vi "tlc_Timing Module Unit Test.vi"() -> ()   [LabVIEW 2010]
uses:
  Controls/tlc_Cue_Information.ctl
  Controls/channel.ctl
  tlc_Timing Module Unit Test States.ctl
  tlc_Timing Command Control.ctl
panel:
  out "Follow Time (s)":dbl format="%.2f"
  out "Fade Time (s)":dbl format="%.2f"
  out "Wait Time (s)":dbl format="%.2f"
  in  "Cue Input":T1 {"Channels"."Intensität" min=0.0 max=100.0 step=1.0 format="%#.0f"}
  # "Measured Test Values"
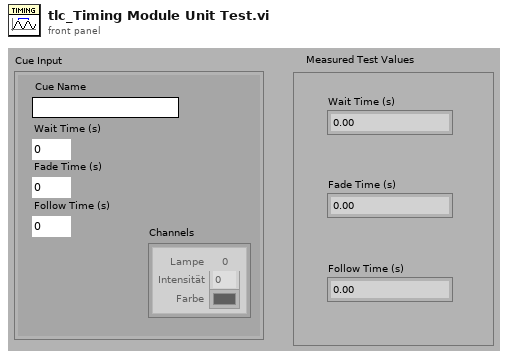
[diagram p1: front panel]
types:
  T1 = typedef "tlc_Cue_Information.ctl" = cluster{"Cue Name":string, "Wait Time (s)":u32, "Fade Time (s)":u32, "Follow Time (s)":u32, "Channels":T2[][]}
  T2 = typedef "channel.ctl" = cluster{"Intensität":dbl, " Farbe":u32, "Channel":i32}
  T3 = typedef "tlc_Timing Module Unit Test States.ctl" = enum16{"Begin Play", "Wait Time", "Fade Time", "Follow Time", "End Play"}
  T4 = typedef "tlc_Timing Command Control.ctl" = enum16{"Start", "Check Time"}
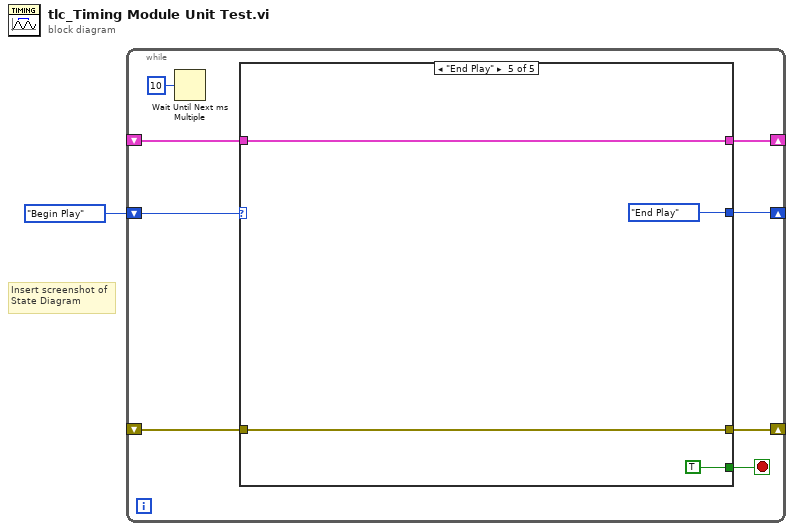
[diagram p0: block diagram]
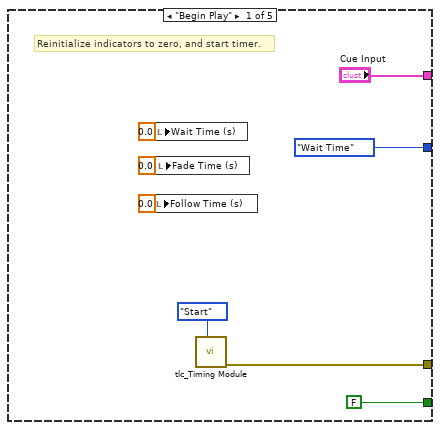
[diagram p2: hidden frame]
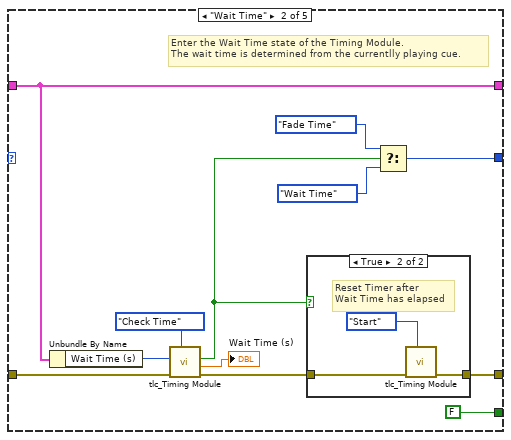
[diagram p3: hidden frame]
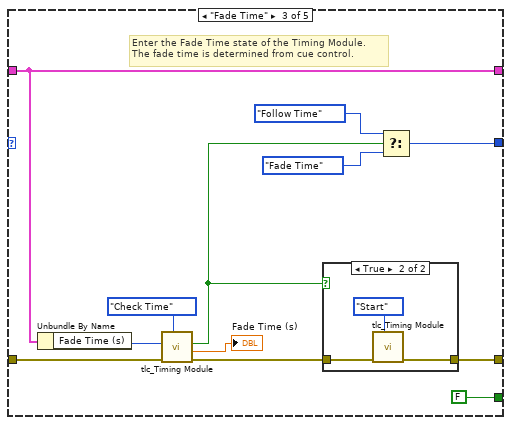
[diagram p5: hidden frame]
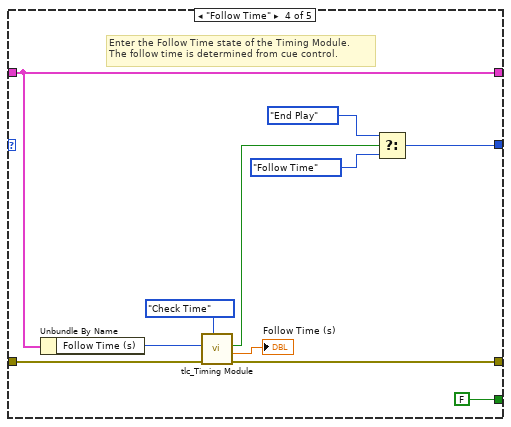
[diagram p7: hidden frame]
diagram:
  # "Insert screenshot of\nState Diagram"
  n1 = while {
    shift-right: [w4] -> _
    shift-left: tlc_Timing_Module_Unit_Test_States."Begin Play" ("tlc_Timing Test States.ctl") -> [w5]
    shift-right: [w8] -> _
    shift-left: _ -> [w9]
    shift-right: [w7] -> _
    shift-left: _ -> [w6]
    stop <- w3 stop-if-true
    # ">Error>"
    n2 = Wait Until Next ms Multiple(millisecond multiple=u32 10) -> ()  [unwired: 1 out]
    n3 = case shown="\"End Play\"" w5 {
      tunnel: [FALSE FALSE FALSE FALSE TRUE] -> w3
      tunnel: w9 -> [_ w27 w42 w60 w62]
      tunnel: [w14 w28 w44 w59 w62] -> w8
      tunnel: [tlc_Timing_Module_Unit_Test_States."Wait Time" ("tlc_Timing Test States.ctl") w22 w43 w52 tlc_Timing_Module_Unit_Test_States."End Play" ("tlc_Timing Test States.ctl")] -> w4
      tunnel: ["Cue Input" w18 w37 w56 w61] -> w7
      tunnel: w6 -> [_ w18 w37 w56 w61]
      frame "Begin Play" {
        # "Reinitialize indicators to zero, and start timer."
        n4 = local write "Follow Time (s)"(0.0 ("Follow Time (s)")) -> ()
        n5 = local write "Wait Time (s)"(0.0 ("Wait Time (s)")) -> ()
        n6 = local write "Fade Time (s)"(0.0 ("Fade Time (s)")) -> ()
        n7 = call "tlc_Timing Module.vi"("Kommando"=tlc_Timing_Command_Control."Start" ("Timer Command")) -> ("error out"=w14:errorcluster)  [unwired: 8 in, 2 out]
      }
      frame "Wait Time" {
        # "Enter the Wait Time state of the Timing Module.\nThe wait time is determined from the currentlly playing cue."
        n8 = Unbundle By Name(w18) -> ("Wait Time (s)"=w23:u32)
        n9 = call "tlc_Timing Module.vi"("Kommando"=tlc_Timing_Command_Control."Check Time" ("Timer Command"), "error in (no error)"=w27, "Ziel Zeit"=w23) -> ("error out"=w26:errorcluster, "Verstrichene Zeit"=→"Wait Time (s)":dbl, "Fertig?"=w25:bool)  [unwired: 6 in]
        n10 = case shown="True" w25 {
          tunnel: w26 -> [w30 w32]
          tunnel: [w30 w33] -> w28
          frame False {
          }
          frame True {
            # "Reset Timer after\nWait Time has elapsed"
            n11 = call "tlc_Timing Module.vi"("Kommando"=tlc_Timing_Command_Control."Start" ("Timer Command"), "error in (no error)"=w32) -> ("error out"=w33:errorcluster)  [unwired: 7 in, 2 out]
          }
        }
        n12 = Select(t=tlc_Timing_Module_Unit_Test_States."Fade Time" ("tlc_Timing Test States.ctl"), s=w25, f=tlc_Timing_Module_Unit_Test_States."Wait Time" ("tlc_Timing Test States.ctl")) -> (s? t:f=w22:T3)
      }
      frame "Fade Time" {
        # "Enter the Fade Time state of the Timing Module.\nThe fade time is determined from cue control."
        n13 = Unbundle By Name(w37) -> ("Fade Time (s)"=w39:u32)
        n14 = call "tlc_Timing Module.vi"("Kommando"=tlc_Timing_Command_Control."Check Time" ("Timer Command"), "error in (no error)"=w42, "Ziel Zeit"=w39) -> ("error out"=w41:errorcluster, "Verstrichene Zeit"=→"Fade Time (s)":dbl, "Fertig?"=w38:bool)  [unwired: 6 in]
        n15 = case shown="True" w38 {
          tunnel: w41 -> [w46 w47]
          tunnel: [w46 w48] -> w44
          frame False {
          }
          frame True {
            n16 = call "tlc_Timing Module.vi"("Kommando"=tlc_Timing_Command_Control."Start" ("Timer Command"), "error in (no error)"=w47) -> ("error out"=w48:errorcluster)  [unwired: 7 in, 2 out]
          }
        }
        n17 = Select(t=tlc_Timing_Module_Unit_Test_States."Follow Time" ("tlc_Timing Test States.ctl"), s=w38, f=tlc_Timing_Module_Unit_Test_States."Fade Time" ("tlc_Timing Test States.ctl")) -> (s? t:f=w43:T3)
      }
      frame "Follow Time" {
        # "Enter the Follow Time state of the Timing Module.\nThe follow time is determined from cue control."
        n18 = Unbundle By Name(w56) -> ("Follow Time (s)"=w57:u32)
        n19 = call "tlc_Timing Module.vi"("Kommando"=tlc_Timing_Command_Control."Check Time" ("Timer Command"), "error in (no error)"=w60, "Ziel Zeit"=w57) -> ("error out"=w59:errorcluster, "Verstrichene Zeit"=→"Follow Time (s)":dbl, "Fertig?"=w53:bool)  [unwired: 6 in]
        n20 = Select(t=tlc_Timing_Module_Unit_Test_States."End Play" ("tlc_Timing Test States.ctl"), s=w53, f=tlc_Timing_Module_Unit_Test_States."Follow Time" ("tlc_Timing Test States.ctl")) -> (s? t:f=w52:T3)
      }
      frame "End Play" {
      }
    }
  }
